vi "Tear Down TS.vi"(8 "error in":errorcluster, 11 "HTS Test Stand in":refnum<class "HTS Test Stand.lvclass">) -> (0 "error out":errorcluster, 3 "HTS Test Stand out":refnum<class "HTS Test Stand.lvclass">)   [LabVIEW 2019, in "Test Stands.lvlib" / "HTS Test Stand.lvclass"]
uses:
  HTS Test Stand.lvclass
  C:/Users/krio/Documents/LV_Projects/test-stand/App/Generic Test Stand/Generic Test Stand.lvclass
  DAC/HTS/Vacum Valve/DAC Vacum Valve.lvclass
  Generic Test Stand/Generic Test Stand.lvclass/Generic Test Stand.ctl
  DAC/DAC.lvclass
  Generic Test Stand/Generic Test Stand.lvclass
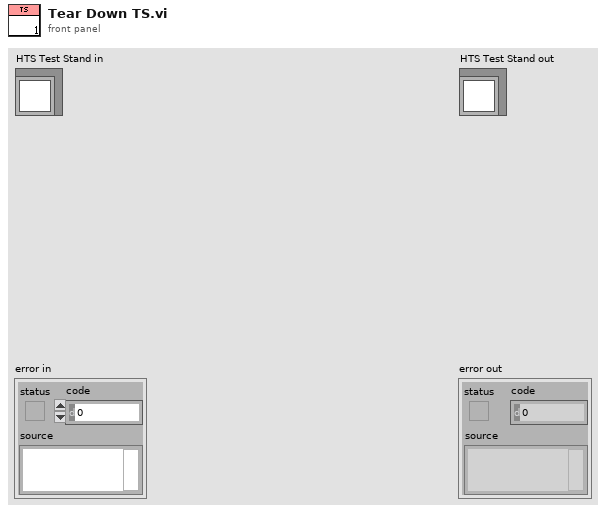
[diagram p1: front panel]
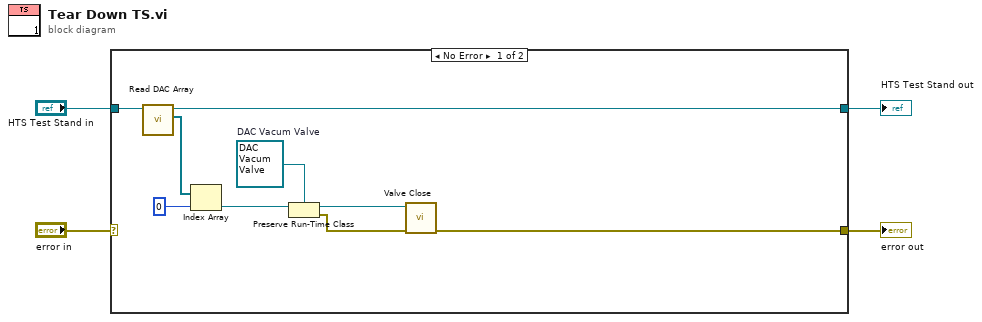
[diagram p0: block diagram]
diagram:
  n1 = case shown="No Error" "error in" {
    selector: "error in" -> [_ w15]
    tunnel: [w7 w15] -> w4
    tunnel: [w9 w14] -> w3
    tunnel: "HTS Test Stand in" -> [w8 w14]
    frame No Error {
      w12 = refnum<class "DAC Vacum Valve.lvclass"> refnum  # DAC Vacum Valve
      n2 = call "Read DAC Array.vi"("Generic Test Stand in"=w8) -> ("DAC Array"=w10:refnum<class "DAC.lvclass">[], "Generic Test Stand out"=w9:refnum<class "HTS Test Stand.lvclass">)  [unwired: 8 in, 1 out]
      n3 = Index Array(array=w10, index=0) -> (element=w13:refnum<class "DAC.lvclass">)
      n4 = Preserve Run-Time Class(object in=w13, 2:w12) -> (object out=w6:refnum<class "DAC Vacum Valve.lvclass">, error out=w5:errorcluster)  [unwired: 1 in]
      n5 = call "Valve Close.vi"("error in (no error)"=w5, "DAC Vacum Valve in"=w6) -> ("error out"=w7:errorcluster)  [unwired: 8 in, 1 out]
    }
    frame Error {
    }
  }
  "error out" <- w4
  "HTS Test Stand out" <- w3
